vi "Destroy XML Editor.vi"(8 "error in (no error)":errorcluster, 11 "Project XML Editor in":refnum<class "Project XML Editor.lvclass">) -> (0 "error out":errorcluster)   [LabVIEW 2018, in ".LVLIBP CD XML Updater.lvlib" / "Project XML Editor.lvclass"]
uses:
  Project XML Editor.lvclass
  Project XML Editor.lvclass/Project XML Editor.ctl
  <vilib>/xml/Close Reference(Node).vi
  <vilib>/xml/NI_XML.lvlib
  <resource>/objmgr/DOMUserDefRef.rc
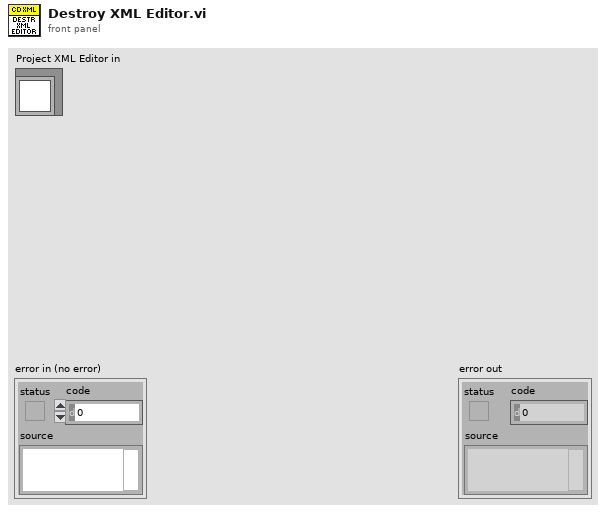
[diagram p1: front panel]
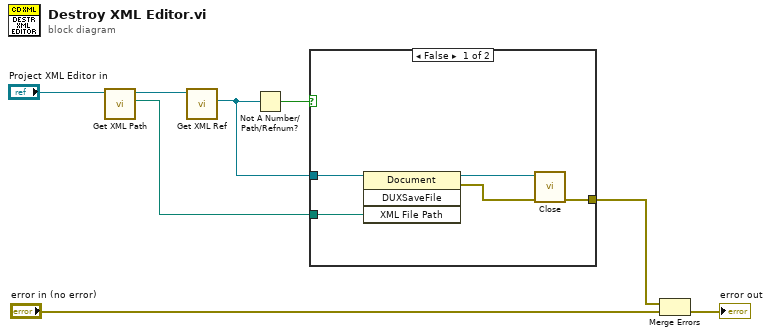
[diagram p0: block diagram]
diagram:
  n1 = call "Get XML Path.vi"("Project XML Editor in"="Project XML Editor in") -> ("XML Path"=w1:path, "Project XML Editor out"=w2:refnum<class "Project XML Editor.lvclass">)  [unwired: 9 in]
  n2 = call "Get XML Ref.vi"("Project XML Editor in"=w2) -> ("XML Ref"=w7:refnum<k20>)  [unwired: 9 in, 1 out]
  n3 = Not A Number/Path/Refnum?(number/path/refnum=w7) -> (NaN/Path/Refnum?=w8:bool)
  n4 = case shown="False" w8 {
    tunnel: w7 -> [w12 _]
    tunnel: [w13 _] -> w5
    tunnel: w1 -> [w9 _]
    frame False {
      n5 = invoke class="Document" method="DUXSaveFile"(reference=w12, "XML File Path"=w9) -> (reference out=w10:refnum<k20>, error out=w11:errorcluster)  [unwired: 2 in, 2 out]
      n6 = call-poly <vilib>:"Close.vi"("error in (no error)"=w11, "node"=w10) -> ("error out"=w13:errorcluster)  [unwired: 7 in]
    }
    frame True {
    }
  }
  n7 = Merge Errors(w5, "error in (no error)") -> (→"error out":errorcluster)
